vi "Log Data DBL.vi"(6 "Identifier":string, 8 "error in":errorcluster, 9 "Time Stamp":timestamp format="%<%x %.3X>T", 10 "Data":dbl, 11 "IDataLogger in":refnum<class "SimpleCsvDataLogger.lvclass">) -> (0 "error out":errorcluster, 3 "IDataLogger out":refnum<class "SimpleCsvDataLogger.lvclass">)   [LabVIEW 2024, in "SimpleCsvDataLogger.lvclass"]
uses:
  SimpleCsvDataLogger.lvclass
  SimpleCsvDataLogger.lvclass/SimpleCsvDataLogger.ctl
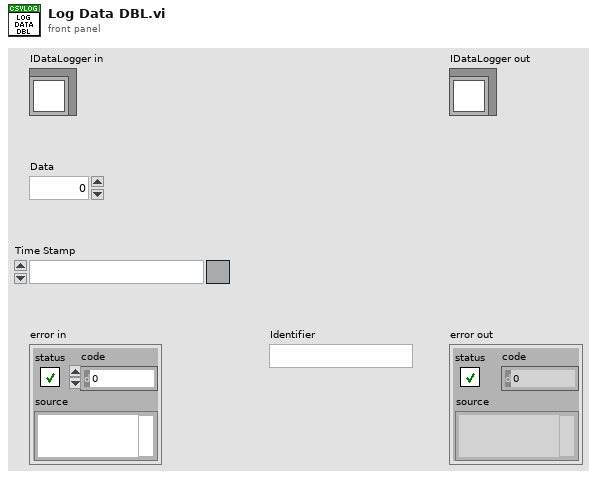
[diagram p1: front panel]
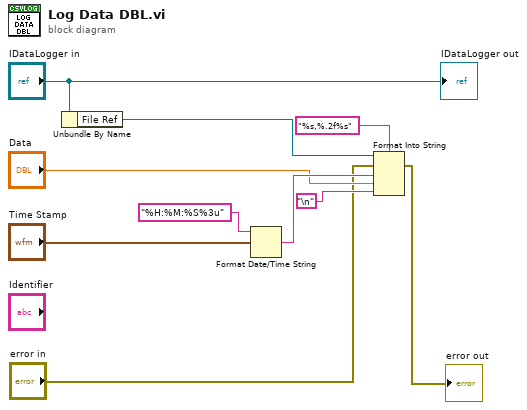
[diagram p0: block diagram]
diagram:
  n1 = Unbundle By Name("IDataLogger in") -> ("File Ref"=w9:refnum<file>)
  n2 = Format Date/Time String(time format string (%c)="%H:%M:%S%3u", seconds (now)="Time Stamp") -> (date/time string=w6:string)  [unwired: 1 in]
  n3 = Format Into String(format string="%s,%.2f%s", initial string=w9, error in="error in", w6, "Data", "\n") -> (error out=→"error out":errorcluster)  [unwired: 1 out]
  "IDataLogger out" <- "IDataLogger in"
